vi "LS370_Calc_Excitation.vi"() -> ()   [LabVIEW 2016]
panel:
  out "text":string[](array[string])
  out "Numeric 2":i32
  in  "Numeric":dbl format="%#_13g"
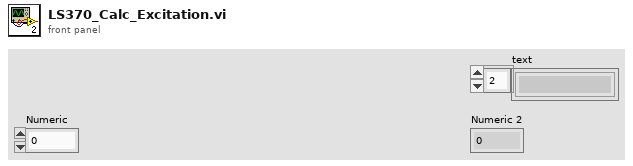
[diagram p1: front panel]
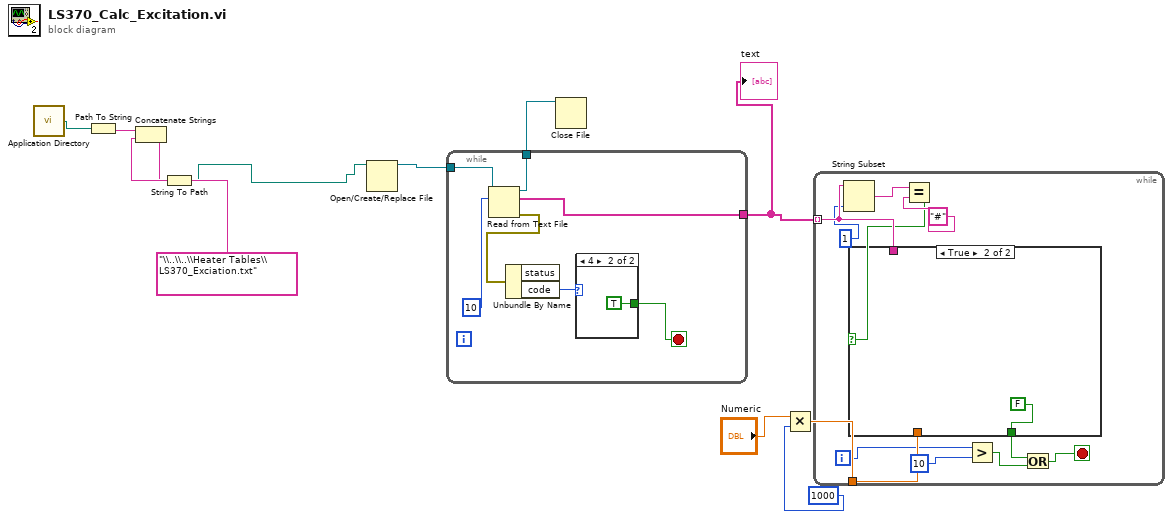
[diagram p0: block diagram]
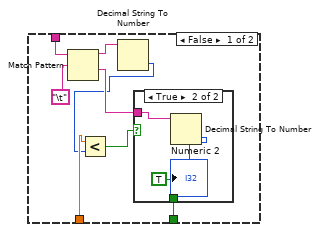
[diagram p2: hidden frame]
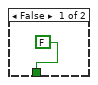
[diagram p3: hidden frame]
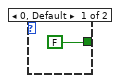
[diagram p4: hidden frame]
diagram:
  n1 = call <vilib>:"Application Directory.vi"() -> ("Application Directory"=w10:path)
  n2 = Path To String(path=w10) -> (string=w8:string)
  n3 = Concatenate Strings(w8, "\\..\\..\\Heater Tables\\LS370_Exciation.txt") -> (w7:string)
  n4 = String To Path(string=w7) -> (path=w6:path)
  n5 = Open/Create/Replace File(file path (use dialog)=w6) -> (refnum out=w11:refnum<file>)  [unwired: 5 in, 2 out]
  n6 = while {
    tunnel: w11 -> [w18]
    tunnel: [w14] -> w1
    tunnel: [w13] -> w2
    stop <- w15 stop-if-true
    n7 = Read from Text File(file (use dialog)=w18, count=10) -> (refnum out=w13:refnum<file>, text=w14:string[], error out=w17:errorcluster)  [unwired: 2 in, 1 out]
    n8 = Unbundle By Name(w17) -> ("code"=w16:i32)  [unwired: 1 out]
    n9 = case shown="4" w16 {
      tunnel: [FALSE TRUE] -> w15
      frame 0, Default {
      }
      frame 4 {
      }
    }
  }
  "text" <- w1
  n10 = Close File(refnum=w2) -> ()  [unwired: 1 in, 2 out]
  n11 = Multiply(x="Numeric", y=1000) -> (x*y=w4:dbl)
  n12 = while {
    tunnel: w1 -> [w30] mode=indexing
    tunnel: w4 -> [w31]
    i -> [w25]
    stop <- w21 stop-if-true
    n13 = String Subset(string=w30, length (rest)=1) -> (substring=w27:string)  [unwired: 1 in]
    n14 = Equal?(x=w27, y="#") -> (x = y?=w26:bool)
    n15 = case shown="True" w26 {
      tunnel: [w35 FALSE] -> w23
      tunnel: w31 -> [w34 _]
      tunnel: w30 -> [w32 _]
      frame False {
        n16 = Match Pattern(string=w32, regular expression="\t") -> (before substring=w38:string, after substring=w37:string)  [unwired: 1 in, 2 out]
        n17 = Decimal String To Number(string=w38) -> (number=w33:i32)  [unwired: 2 in, 1 out]
        n18 = Less?(x=w34, y=w33) -> (x < y?=w36:bool)
        n19 = case shown="True" w36 {
          tunnel: w37 -> [_ w43]
          tunnel: [FALSE TRUE] -> w35
          frame False {
          }
          frame True {
            n20 = Decimal String To Number(string=w43) -> (number=→"Numeric 2":i32)  [unwired: 2 in, 1 out]
          }
        }
      }
      frame True {
      }
    }
    n21 = Greater?(x=w25, y=10) -> (0:w22:bool)
    n22 = Or(x=w23, y=w22) -> (x .or. y?=w21:bool)
  }
